vi "Import Custom Device (New).vi"(8 "error in":errorcluster, 9 "name":string, 10 "path":path, 11 "custom devices ref in":T1 format="%.0x") -> (0 "error out":errorcluster, 2 "custom device ref":T1 format="%.0x", 3 "custom devices ref out":T1 format="%.0x")   [LabVIEW 2020, in "AIM MIL-STD-1553 Scripting.lvlib"]
uses:
  AIM MIL-STD-1553 Scripting.lvlib
  <vilib>/NI/VeriStand Custom Device Serialization/Custom Device Serialization.lvlib
  <vilib>/NI/VeriStand Custom Device Serialization/Import as Child.vi
  <vilib>/NI VeriStand/Custom Device API/Custom Device Item Ref.ctl
  <vilib>/NI VeriStand/Custom Device API/Custom Device API.lvlib
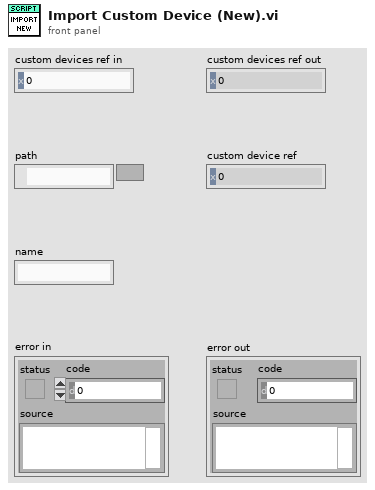
[diagram p1: front panel]
types:
  T1 = typedef "Custom Device API.lvlib/Custom Device Item Ref.ctl" = u64
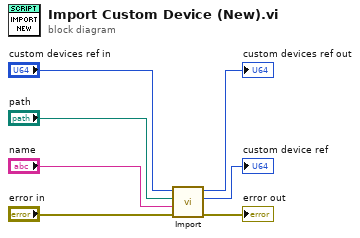
[diagram p0: block diagram]
diagram:
  n1 = call-poly <vilib>:"Import.vi"("error in"="error in", "name"="name", "path"="path", "parent ref in"="custom devices ref in") -> ("error out"=→"error out":errorcluster, "new item ref"=→"custom device ref":T1, "parent ref out"=→"custom devices ref out":T1)  [unwired: 5 in]
